vi "HR_Zones_Format_Levels.vi"(8 "error in (no error)":errorcluster, 11 "HR Data Structure":T1) -> (0 "error out":errorcluster, 3 "HR Data Structure 2":T1)   [LabVIEW 2021]
doc: "This Vi creates %HR MAX levels and writes it into array in data cluster"
uses:
  Controls/HR Data Structure.ctl
  Controls/Runner's Data.ctl
  Controls/Raw Data.ctl
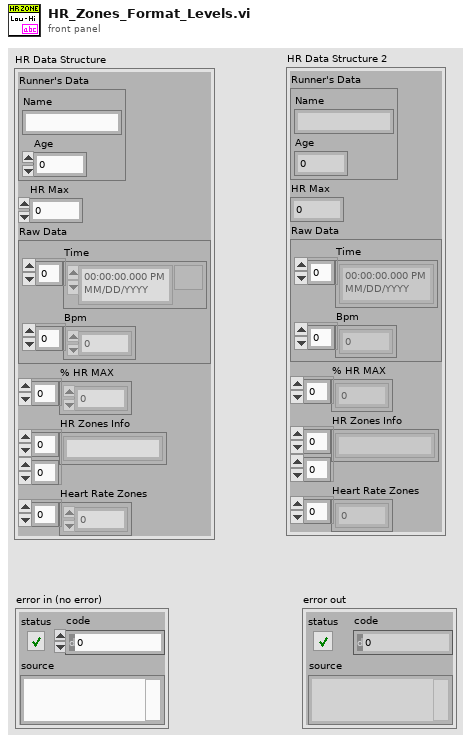
[diagram p1: front panel]
types:
  T1 = typedef "HR Data Structure.ctl" = cluster{"Runner's Data":T2, "HR Max":i32, "Raw Data":T3, "% HR MAX ":dbl[], "HR Zones Info":string[][], "Heart Rate Zones":dbl[]}
  T2 = typedef "Runner's Data.ctl" = cluster{"Name":string, "Age":i32}
  T3 = typedef "Raw Data.ctl" = cluster{"Time":timestamp[], "Bpm":i32[]}
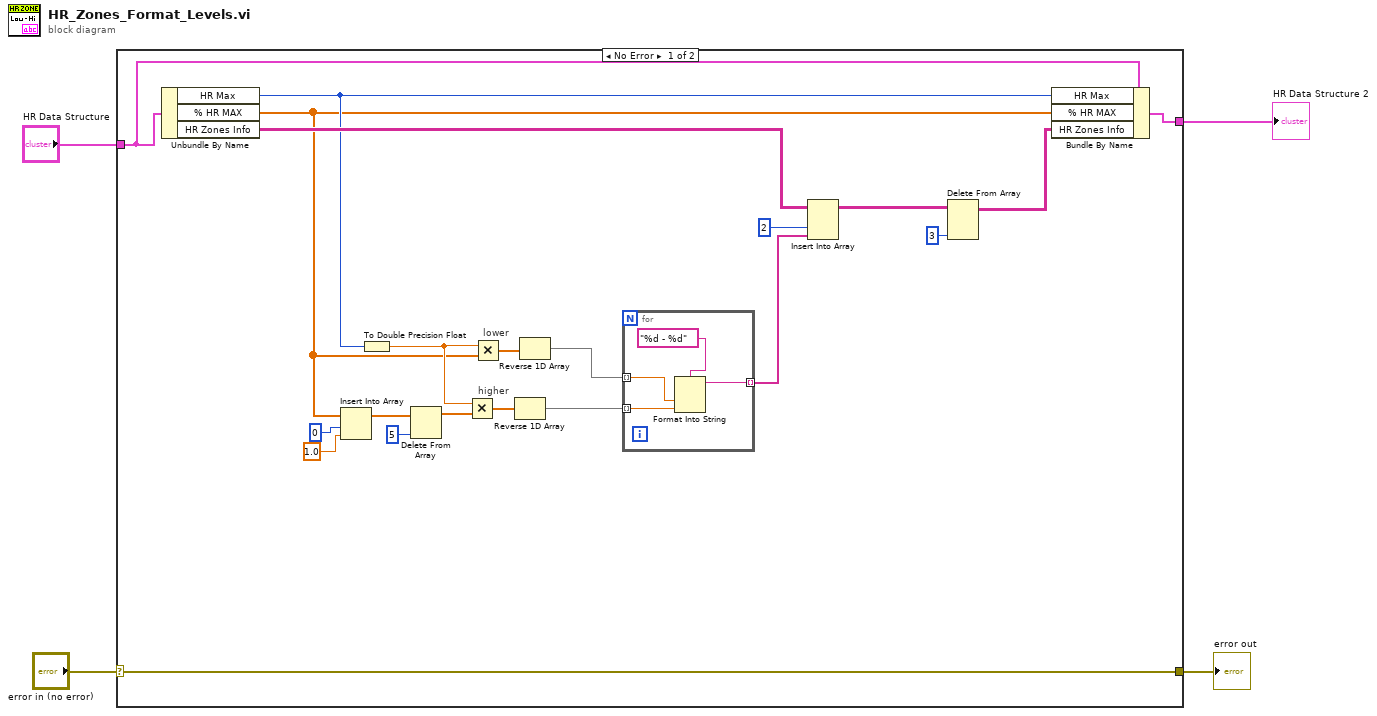
[diagram p0: block diagram]
diagram:
  n1 = case shown="No Error" "error in (no error)" {
    selector: "error in (no error)" -> [w13 w31]
    tunnel: "HR Data Structure" -> [w12 w30]
    tunnel: [w13 w31] -> w2
    tunnel: [w11 w30] -> w1
    frame No Error {
      # "higher"
      # "lower"
      n2 = Unbundle By Name(w12) -> ("HR Max"=w10:i32, "% HR MAX"=w9:dbl[], "HR Zones Info"=w25:string[][])
      n3 = Insert Into Array(array=w9, index=0, new element=1.0) -> (w16:dbl[])
      n4 = To Double Precision Float(number=w10) -> (double precision float=w23:dbl)
      n5 = Delete From Array(array=w16, index=5) -> (array with subset deleted=w19:dbl[])  [unwired: 1 in, 1 out]
      n6 = Multiply(x=w23, y=w19) -> (x*y=w21:dbl[])
      n7 = Multiply(x=w23, y=w9) -> (x*y=w22:dbl[])
      n8 = Reverse 1D Array(array=w21) -> (reversed array=w20:dbl[])
      n9 = Reverse 1D Array(array=w22) -> (reversed array=w18:dbl[])
      n10 = for {
        tunnel: w18 -> [w29] mode=indexing
        tunnel: [w27] -> w24 mode=indexing
        tunnel: w20 -> [w26] mode=indexing
        n11 = Format Into String(format string="%d - %d", w29, w26) -> (resulting string=w27:string)  [unwired: 2 in, 1 out]
      }
      n12 = Insert Into Array(array=w25, index (col)=2, new element=w24) -> (w7:string[][])  [unwired: 1 in]
      n13 = Delete From Array(array=w7, index (col)=3 ("disabled index (col)")) -> (array with subset deleted=w6:string[][])  [unwired: 2 in, 1 out]
      n14 = Bundle By Name(cluster=w12, "HR Max"=w10, "% HR MAX"=w9, "HR Zones Info"=w6) -> (w11:T1)
    }
    frame Error {
    }
  }
  "error out" <- w2
  "HR Data Structure 2" <- w1
